vi "get_file_sent.vi"(8 "error in (no error)":errorcluster, 10 "path array in":path[](array[path]), 11 "ErrorController in":refnum<class "ErrorController.lvclass">) -> (0 "error out":errorcluster, 2 "path array out":path[](array[path]), 3 "ErrorController out":refnum<class "ErrorController.lvclass">)   [LabVIEW 2010, in "ErrorController.lvclass"]
uses:
  ErrorController.lvclass
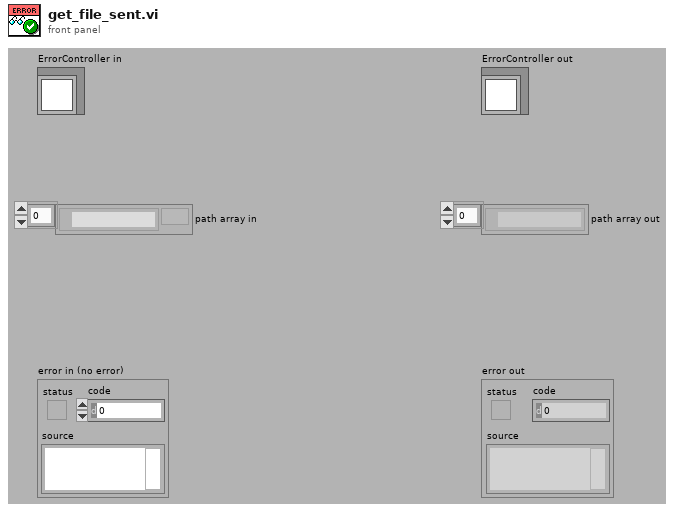
[diagram p1: front panel]
types:
  T1 = enum16{"open", "replace", "create", "open or create", "replace or create", "replace or create with confirmation"}
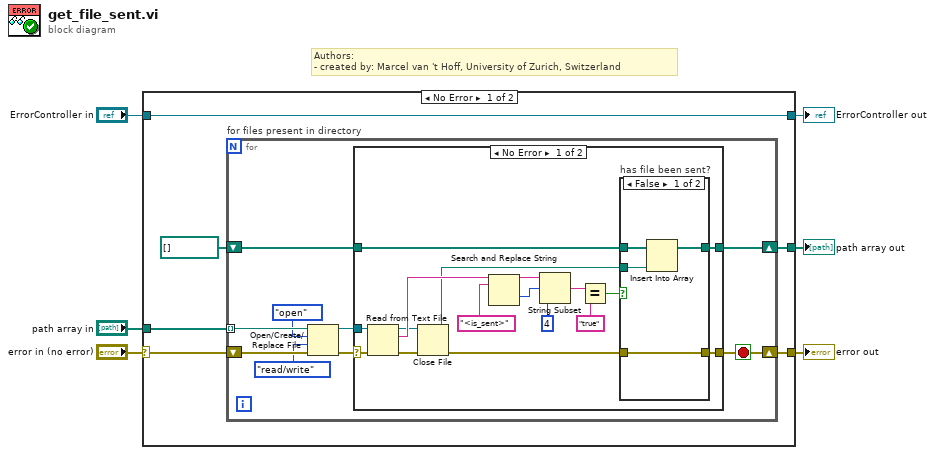
[diagram p0: block diagram]
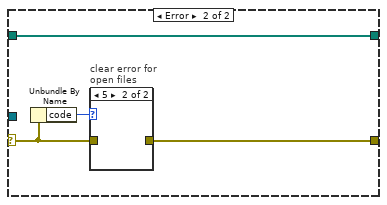
[diagram p3: hidden frame]
diagram:
  # "Authors: \n- created by: Marcel van 't Hoff, University of Zurich, Switzerland"
  n1 = case shown="No Error" "error in (no error)" {
    selector: "error in (no error)" -> [w7 w52]
    tunnel: [w11 w52] -> w5
    tunnel: [w12 w51] -> w3
    tunnel: "ErrorController in" -> [w12 w51]
    tunnel: [w9 w50] -> w1
    tunnel: "path array in" -> [w8 w50]
    frame No Error {
      n2 = for "for files present in directory" {
        tunnel: w8 -> [w21] mode=indexing
        shift-right: [w14] -> w11
        shift-left: w7 -> [w19]
        shift-right: [w15] -> w9
        shift-left: path[] [] -> [w16]
        stop <- w14 stop-if-true
        n3 = Open/Create/Replace File(file path (use dialog)=w21, error in=w19, operation (0:open)=T1."open", access (0:read/write)=enum16{"read/write", "read-only", "write-only"}."read/write") -> (refnum out=w20:refnum<file>, error out=w13:errorcluster)  [unwired: 2 in, 1 out]
        n4 = case shown="No Error" w13 {
          selector: w13 -> [w22 w45]
          tunnel: w20 -> [w38 _]
          tunnel: w16 -> [w37 w48]
          tunnel: [w36 w48] -> w15
          tunnel: [w27 w46] -> w14
          frame No Error {
            n5 = Read from Text File(file (use dialog)=w38, error in=w22) -> (refnum out=w26:refnum<file>, text=w31:string, error out=w24:errorcluster)  [unwired: 2 in, 1 out]
            n6 = Close File(refnum=w26, error in=w24) -> (path=w25:path, error out=w23:errorcluster)
            n7 = Search and Replace String(input string=w31, search string="<is_sent>") -> (result string=w30:string, offset past replacement=w28:i32)  [unwired: 6 in, 2 out]
            n8 = String Subset(string=w30, offset (0)=w28, length (rest)=4 ("length (rest)")) -> (substring=w35:string)
            n9 = Equal?(x=w35, y="true") -> (x = y?=w33:bool)
            n10 = case "has file been sent?" shown="False" w33 {
              tunnel: w25 -> [w41 _]
              tunnel: w37 -> [w42 w44]
              tunnel: [w40 w44] -> w36
              tunnel: w23 -> [w39 w43]
              tunnel: [w39 w43] -> w27
              frame False {
                n11 = Insert Into Array(array=w42, new element=w41) -> (w40:path[])  [unwired: 1 in]
              }
              frame True {
              }
            }
          }
          frame Error {
            n12 = Unbundle By Name(w45) -> ("code"=w47:i32)
            n13 = case "clear error for\nopen files" shown="5" w47 {
              tunnel: [w49 _] -> w46
              tunnel: w45 -> [w49 _]
              frame Default {
              }
              frame 5 {
              }
            }
          }
        }
      }
    }
    frame Error {
    }
  }
  "error out" <- w5
  "ErrorController out" <- w3
  "path array out" <- w1
